vi "Build 1D Array.vi"(0 "Channel Data":T1, 11 "Error In":errorcluster) -> (4 "U8 Array":u8[](array[numeric]), 15 "Error Out":errorcluster)   [LabVIEW 2021]
doc: "This VI builds the 1D U8 array from U8 array obtained from different channels along with flags."
uses:
  Controls/Channel Data.ctl
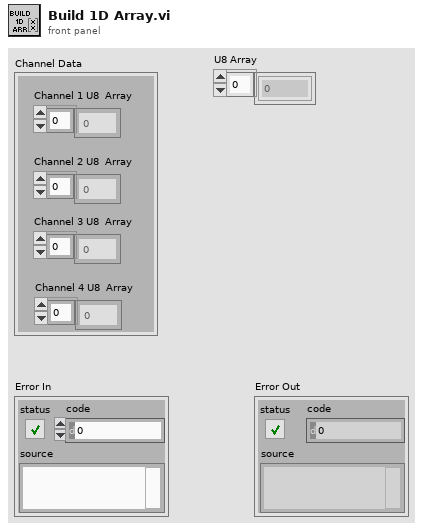
[diagram p1: front panel]
types:
  T1 = typedef "Channel Data.ctl" = cluster{"Channel 1 U8  Array":u8[], "Channel 2 U8  Array ":u8[], "Channel 3 U8  Array":u8[], "Channel 4 U8  Array":u8[]}
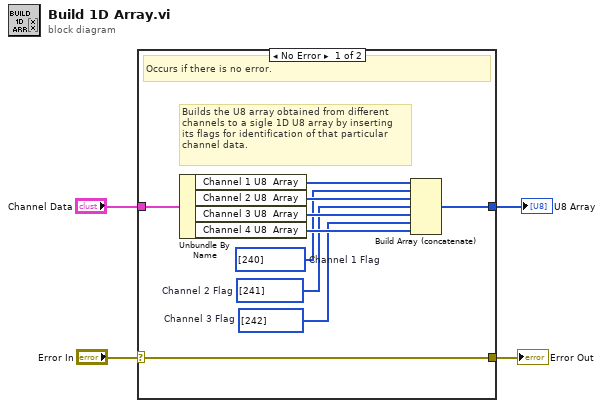
[diagram p0: block diagram]
diagram:
  n1 = case shown="No Error" "Error In" {
    selector: "Error In" -> [w5 w15]
    tunnel: "Channel Data" -> [w14 _]
    tunnel: [w6 _] -> w3
    tunnel: [w5 w15] -> w1
    frame No Error {
      w7 = u8[] [242]  # Channel 3 Flag
      w8 = u8[] [241]  # Channel 2 Flag
      w9 = u8[] [240]  # Channel 1 Flag
      # "Builds the U8 array obtained from different \nchannels to a sigle 1D U8 array by inserting\nits flags for identification of that particular \nchannel data."
      # "Occurs if there is no error."
      n2 = Unbundle By Name(w14) -> ("Channel 1 U8  Array"=w13:u8[], "Channel 2 U8  Array"=w12:u8[], "Channel 3 U8  Array"=w11:u8[], "Channel 4 U8  Array"=w10:u8[])
      n3 = Build Array (concatenate)(w13, w9, w12, w8, w11, w7, w10) -> (w6:u8[])
    }
    frame Error {
      # "Occurs if there is any error"
    }
  }
  "Error Out" <- w1
  "U8 Array" <- w3
